vi "Configure Recorder Output Scaling.vi"(8 "error in (no error)":errorcluster, 9 "Recorder Upper Limit (20)":dbl=20.0, 10 "Recorder Lower Limit (-150)":dbl=-150.0, 11 "VISA resource name":refnum<visa-resource-name>) -> (0 "error out":errorcluster, 3 "VISA resource name out":refnum<visa-resource-name>)   [LabVIEW 2018, in "Agilent U2000 Series.lvlib"]
doc: "Sets the scaling value for the recorder output.\n\nNote: \nThis VI is not applicable for U2040 X-Series."
uses:
  Agilent U2000 Series.lvlib
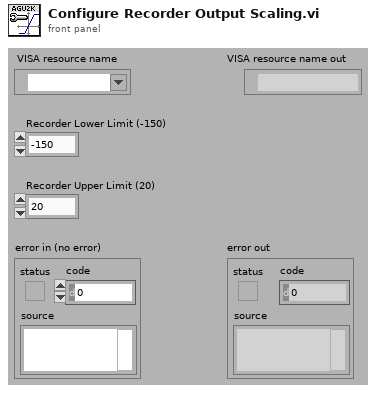
[diagram p1: front panel]
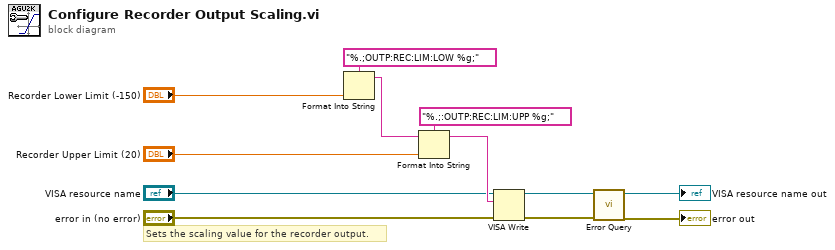
[diagram p0: block diagram]
diagram:
  # "Sets the scaling value for the recorder output."
  n1 = Format Into String(format string="%.;OUTP:REC:LIM:LOW %g;", "Recorder Lower Limit (-150)") -> (resulting string=w10:string)  [unwired: 2 in, 1 out]
  n2 = Format Into String(format string="%.;:OUTP:REC:LIM:UPP %g;", initial string=w10, "Recorder Upper Limit (20)") -> (resulting string=w7:string)  [unwired: 1 in, 1 out]
  n3 = VISA Write(VISA resource name="VISA resource name", write buffer=w7, error in (no error)="error in (no error)") -> (VISA resource name out=w4:refnum<visa-resource-name>, error out=w3:errorcluster)  [unwired: 1 out]
  n4 = call "Error Query.vi"("error in (no error)"=w3, "VISA resource name"=w4) -> ("error out"=→"error out":errorcluster, "VISA resource name out"=→"VISA resource name out":refnum<visa-resource-name>)  [unwired: 8 out]
